vi "Execute.vi"(8 "error in":errorcluster, 11 "O3 Flow Rate Step in":refnum<class "MFC Cell 2 Rate Step.lvclass">) -> (0 "error out":errorcluster, 1 "Next Step?":bool, 2 "MSG":string, 3 "O3 Flow Rate Step out":refnum<class "MFC Cell 2 Rate Step.lvclass">)   [LabVIEW 2017, in "Controller.lvlib" / "MFC Cell 2 Rate Step.lvclass"]
uses:
  MFC Cell 2 Rate Step.lvclass
  C:/Program Files (x86)/National Instruments/LabVIEW 2017/vi.lib/MSR Consulting, LLC/General Reuse/Sequence/STEPS/LEAVES/Double/Switch DBL.lvclass
  <vilib>/MSR Consulting, LLC/General Reuse/Sequence/STEPS/LEAVES/Double/Switch DBL.lvclass/Switch DBL.ctl
  Messages/Update Ctl Device Setpoint MSG/Update Ctl Device Setpoint MSG.lvclass
  C:/Program Files (x86)/National Instruments/LabVIEW 2017/vi.lib/ActorFramework/Message/Message.lvclass
  Messages/Update Ctl Device Setpoint MSG/Update Ctl Device Setpoint MSG.lvclass/Update Ctl Device Setpoint MSG.ctl
  <vilib>/ActorFramework/Message Enqueuer/Message Enqueuer.lvclass/Message Enqueuer.ctl
  Messages/Update Ctl Device Setpoint MSG/Write device.vi
  Messages/Update Ctl Device Setpoint MSG/Write sp.vi
  <vilib>/MSR Consulting, LLC/General Reuse/Sequence/STEPS/LEAVES/Double/Read val.vi
  <vilib>/ActorFramework/Message Priority Queue/Priority Enqueue.vi
  gController.lvclass
  <vilib>/ActorFramework/Message Enqueuer/Message Enqueuer.lvclass
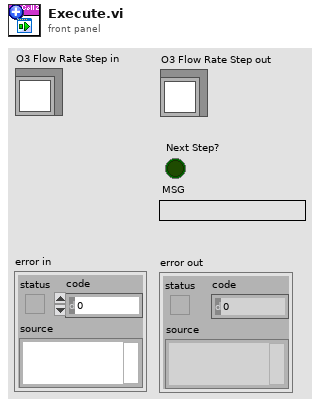
[diagram p1: front panel]
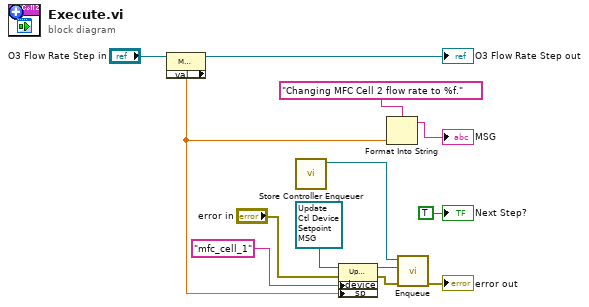
[diagram p0: block diagram]
diagram:
  n1 = property class="MFC Cell 2 Rate Step.lvclass"(reference="O3 Flow Rate Step in") -> (reference out=→"O3 Flow Rate Step out":refnum<class "MFC Cell 2 Rate Step.lvclass">, "val"=w1:dbl)  [unwired: 1 in, 1 out]
  n2 = call "Store Controller Enqueuer.vi"() -> ("Controller Enqueuer Out"=w9:refnum<class "Message Enqueuer.lvclass">)  [unwired: 11 in]
  n3 = property class="Update Device Setpoint MSG"(reference=refnum<class "Update Ctl Device Setpoint MSG.lvclass"> refnum ("Controller.lvlib:Update Device Setpoint MSG"), error in="error in", "device"="mfc_cell_1", "sp"=w1) -> (reference out=w10:refnum<class "Update Ctl Device Setpoint MSG.lvclass">, error out=w6:errorcluster)
  n4 = Format Into String(format string="Changing MFC Cell 2 flow rate to %f.", w1) -> (resulting string=→"MSG":string)  [unwired: 2 in, 1 out]
  n5 = call <vilib>:"Enqueue.vi"("error in (no error)"=w6, "Message"=w10, "Message Enqueuer in"=w9) -> ("error out"=→"error out":errorcluster)  [unwired: 7 in, 1 out]
  "Next Step?" <- TRUE ("Next Step?")
